vi "Configure Sense Connection.vi"(8 "error in (no error)":errorcluster, 9 "Sense Mode (0: Local Sense)":i32(ring) items=["Local Sense", "Remote Sense"], 10 "Source Measure Unit Channel (0: Channel A)":i32(ring) items=["Channel A", "Channel B"], 11 "VISA resource name":refnum<visa-resource-name>) -> (0 "error out":errorcluster, 3 "VISA resource name out":refnum<visa-resource-name>)   [LabVIEW 2019, in "Keithley 2600 Series.lvlib"]
doc: "Configures the state of the sense mode."
uses:
  Keithley 2600 Series.lvlib
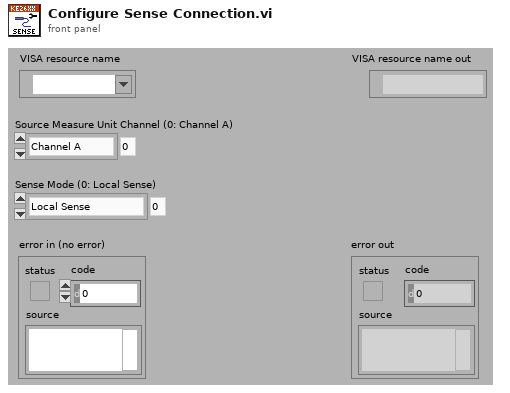
[diagram p1: front panel]
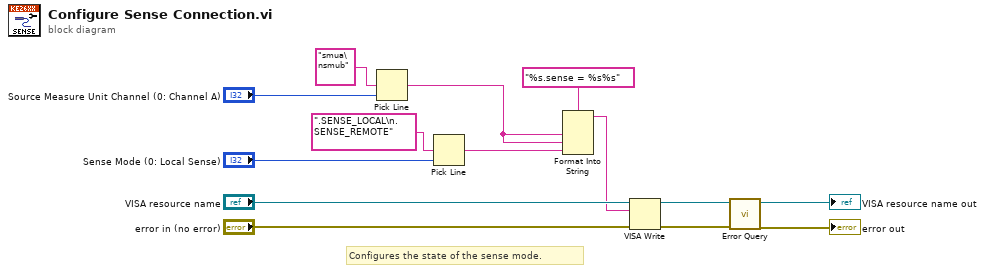
[diagram p0: block diagram]
diagram:
  # "Configures the state of the sense mode."
  n1 = Pick Line(multi-line string="smua\nsmub", line index="Source Measure Unit Channel (0: Channel A)") -> (output string=w9:string)  [unwired: 1 in]
  n2 = Pick Line(multi-line string=".SENSE_LOCAL\n.SENSE_REMOTE", line index="Sense Mode (0: Local Sense)") -> (output string=w8:string)  [unwired: 1 in]
  n3 = Format Into String(format string="%s.sense = %s%s", w9, w9, w8) -> (resulting string=w1:string)  [unwired: 2 in, 1 out]
  n4 = VISA Write(VISA resource name="VISA resource name", write buffer=w1, error in (no error)="error in (no error)") -> (VISA resource name out=w5:refnum<visa-resource-name>, error out=w4:errorcluster)  [unwired: 1 out]
  n5 = call "Error Query.vi"("error in (no error)"=w4, "VISA resource name"=w5) -> ("error out"=→"error out":errorcluster, "VISA resource name out"=→"VISA resource name out":refnum<visa-resource-name>)  [unwired: 6 in, 2 out]
